vi "Set Freq Correction.vi"(8 "error in (no error)":errorcluster, 10 "Frequency Correction (ppm)":i32, 11 "RTL-SDR in":refnum<class "RTL-SDR.lvclass">) -> (0 "error out":errorcluster, 1 "function return":i32, 3 "RTL-SDR out":refnum<class "RTL-SDR.lvclass">)   [LabVIEW 2015, in "RTL-SDR.lvclass"]
doc: "Created IvanLis by LabVIEW Portal\nProfile: http://labviewportal.org/memberlist.php?mode=viewprofile&u=987\neMail: IvanLisanov@gMail.com\nTelegram: https://t.me/IvanLis"
uses:
  RTL-SDR.lvclass
  RTL-SDR.lvclass/RTL-SDR.ctl
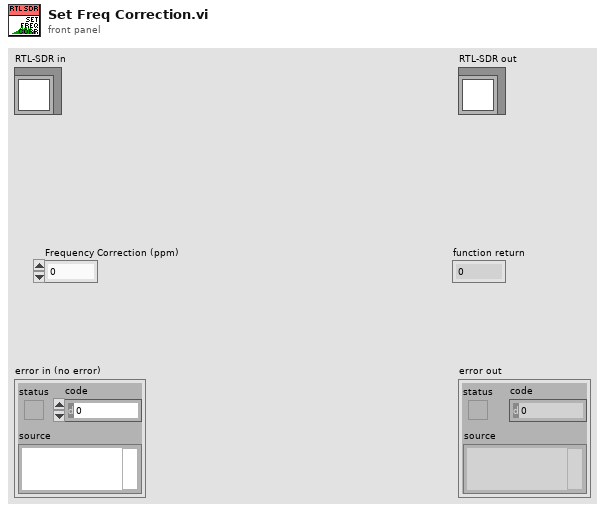
[diagram p1: front panel]
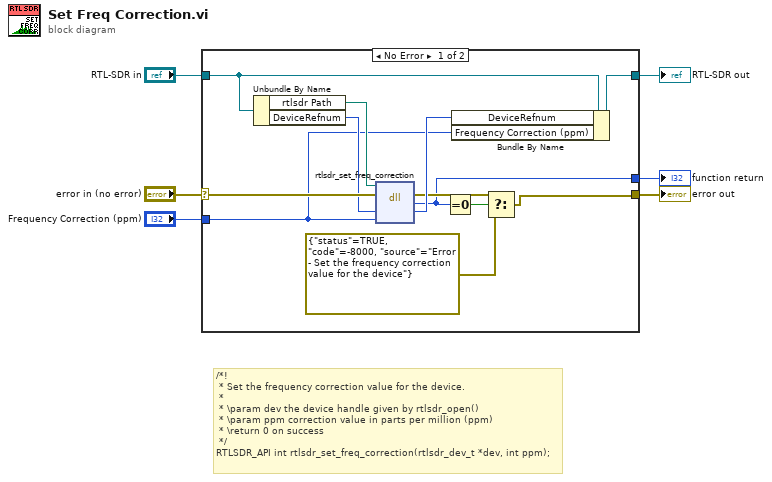
[diagram p0: block diagram]
diagram:
  # "/*!\n * Set the frequency correction value for the device.\n *\n * \\param dev the device handle given by rtlsdr_open()\n * \\param ppm correction value in parts per million (ppm)\n * \\return 0 on success\n */\nRTLSDR_API int rtlsdr_set_freq_correction(rtlsdr_dev_t *dev, int ppm);"
  n1 = case shown="No Error" "error in (no error)" {
    selector: "error in (no error)" -> [w18 w20]
    tunnel: [w8 w20] -> w5
    tunnel: [w16 w19] -> w3
    tunnel: "RTL-SDR in" -> [w17 w19]
    tunnel: [w9 _] -> w2
    tunnel: "Frequency Correction (ppm)" -> [w12 _]
    frame No Error {
      n2 = Unbundle By Name(w17) -> ("rtlsdr Path"=w13:path, "DeviceRefnum"=w15:u64)
      n3 = dll-call lib="C:/Users/Ivan/Desktop/D-23-09-24 (RTL-SDR)/Project (Pelleng-SDR)/RTL-SDR Class/dll/rtlsdr.*" fn="rtlsdr_set_freq_correction"(path in=w13, error in=w18, "DeviceRefnum"=w15, "Frequency Correction (ppm)"=w12) -> (error out=w10:errorcluster, "return type"=w9:i32, "DeviceRefnum"=w14:u64)  [unwired: 2 in, 1 out]
      n4 = Equal To 0?(x=w9) -> (x = 0?=w11:bool)
      n5 = Bundle By Name(cluster=w17, "DeviceRefnum"=w14, "Frequency Correction (ppm)"=w12) -> (w16:refnum<class "RTL-SDR.lvclass">)
      n6 = Select(t=w10, s=w11, f=errorcluster {"status"=TRUE, "code"=-8000, "source"="Error - Set the frequency correction value for the device"} ("error out")) -> (s? t:f=w8:errorcluster)
    }
    frame Error {
    }
  }
  "error out" <- w5
  "RTL-SDR out" <- w3
  "function return" <- w2
